vi "Sub_FFT.vi"(8 "Bound to 1st Frequency":bool=TRUE, 9 "Frequency Method":T2(ring), 10 "Accelerometer sample":dbl[](array[numeric]), 11 "Experiment":T1) -> (0 "Low-Energy Warning":bool, 1 "Frequency measured":dbl, 2 "FFT":dbl[](array[numeric]), 3 "ACC Data":dbl[](array[numeric]))   [LabVIEW 2021]
uses:
  <vilib>/Analysis/4window.llb/Hanning Window (DBL).vi
  <vilib>/Analysis/5stat.llb/RMS (DBL).vi
  <vilib>/Analysis/4window.llb/Hamming Window (DBL).vi
  <vilib>/Analysis/2dsp.llb/Real FFT.vi
  <vilib>/Analysis/4window.llb/AllCosWindow (DBL).vi
  <vilib>/addons/Time Series Analysis/Series Preprocess.llb/TSA Moving Average (Array).vi
  <vilib>/measure/maresamp.llb/Resample Waveform (continuous).vi
  <vilib>/Analysis/NI_AALPro.lvlib
  <vilib>/addons/_Advanced Signal Processing/NI_AdvSigProcTSA.lvlib
  <vilib>/measure/NI_MAPro.lvlib
panel:
  in  "Frequency selection method":T3(ring)
  in  "Use Top N freq components":i32=5 min=1 max=50 step=1
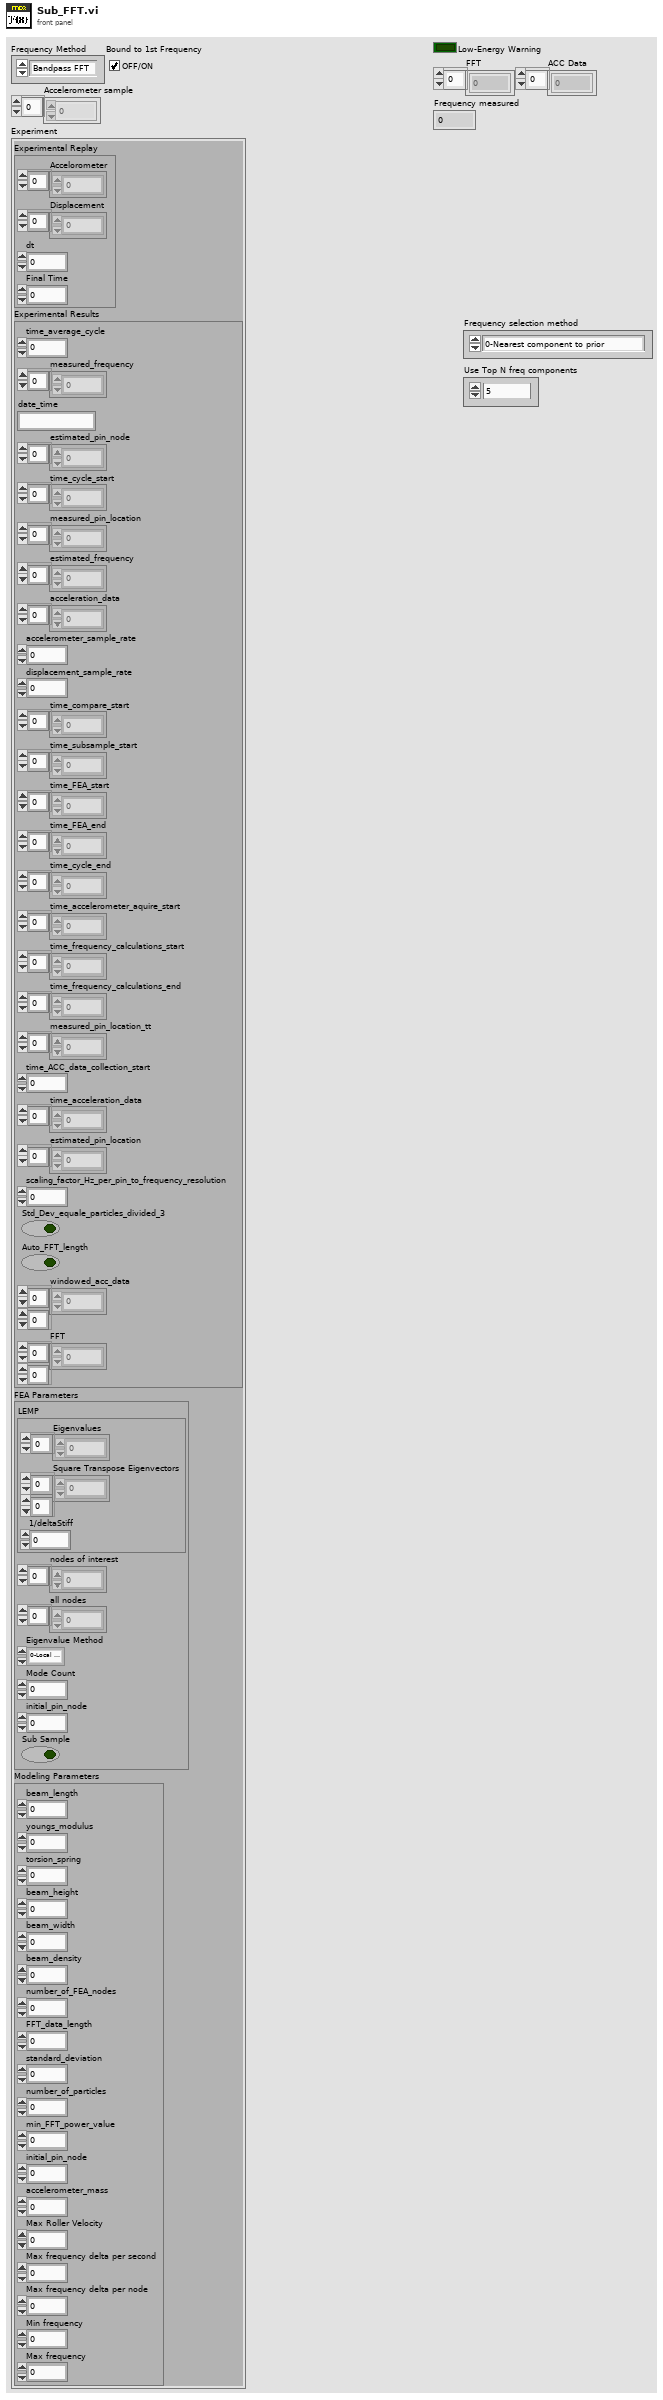
[diagram p1: front panel]
types:
  T1 = cluster{"Experimental Replay":cluster{"Accelorometer":dbl[], "Displacement":dbl[], "dt":dbl, "Final Time":dbl}, "Experimental Results":cluster{"time_average_cycle":dbl, "measured_frequency":dbl[], "date_time":string, "estimated_pin_node":i32[], "time_cycle_start":dbl[], "measured_pin_location":dbl[], "estimated_frequency":dbl[], "acceleration_data":dbl[], "accelerometer_sample_rate":dbl, "displacement_sample_rate":dbl, "time_compare_start":dbl[], "time_subsample_start":dbl[], "time_FEA_start":dbl[], "time_FEA_end":dbl[], "time_cycle_end":dbl[], "time_accelerometer_aquire_start":dbl[], "time_frequency_calculations_start":dbl[], "time_frequency_calculations_end":dbl[], "measured_pin_location_tt":dbl[], "time_ACC_data_collection_start":dbl, "time_acceleration_data":dbl[], "estimated_pin_location":dbl[], "scaling_factor_Hz_per_pin_to_frequency_resolution":dbl, "Std_Dev_equale_particles_divided_3":bool, "Auto_FFT_length":bool, "windowed_acc_data":dbl[][], "FFT":dbl[][]}, "FEA Parameters":cluster{"LEMP":cluster{"Eigenvalues":dbl[], "Square Transpose Eigenvectors":dbl[][], "1/deltaStiff":dbl}, "nodes of interest":i32[], "all nodes":i32[], "Eigenvalue Method":enum16{"0-Local Eigen Modification Procedure", "1-LabVIEW generalized eigenvalues", "2-LabVIEW M^-1K eigenvalues", "3-LabVIEW Cholesky Factorization", "4-Cholesky Factorization CPU SGL", "5-Cholesky Factorization CPU FXP", "6-Cholesky Factorization FPGA SGL", "7-Cholesky Factorization FPGA SGL SCL"}, "Mode Count":i32, "initial_pin_node":i32, "Sub Sample":bool}, "Modeling Parameters":cluster{"beam_length":dbl, "youngs_modulus":dbl, "torsion_spring":dbl, "beam_height":dbl, "beam_width":dbl, "beam_density":dbl, "number_of_FEA_nodes":i32, "FFT_data_length":i32, "standard_deviation":dbl, "number_of_particles":i32, "min_FFT_power_value":dbl, "initial_pin_node":i32, "accelerometer_mass":dbl, "Max Roller Velocity":dbl, "Max frequency delta per second":dbl, "Max frequency delta per node":dbl, "Min frequency":dbl, "Max frequency":dbl}}
  T2 = enum16{"Bandpass FFT", "Tone", "FFT", "Custom Filter"}
  T3 = enum16{"0-Nearest component to prior ", "1-Coerce maximum differential", "2-Average with nearest component", "3-Top by power", "4-Lowest major component", "5-Average with lowest component"}
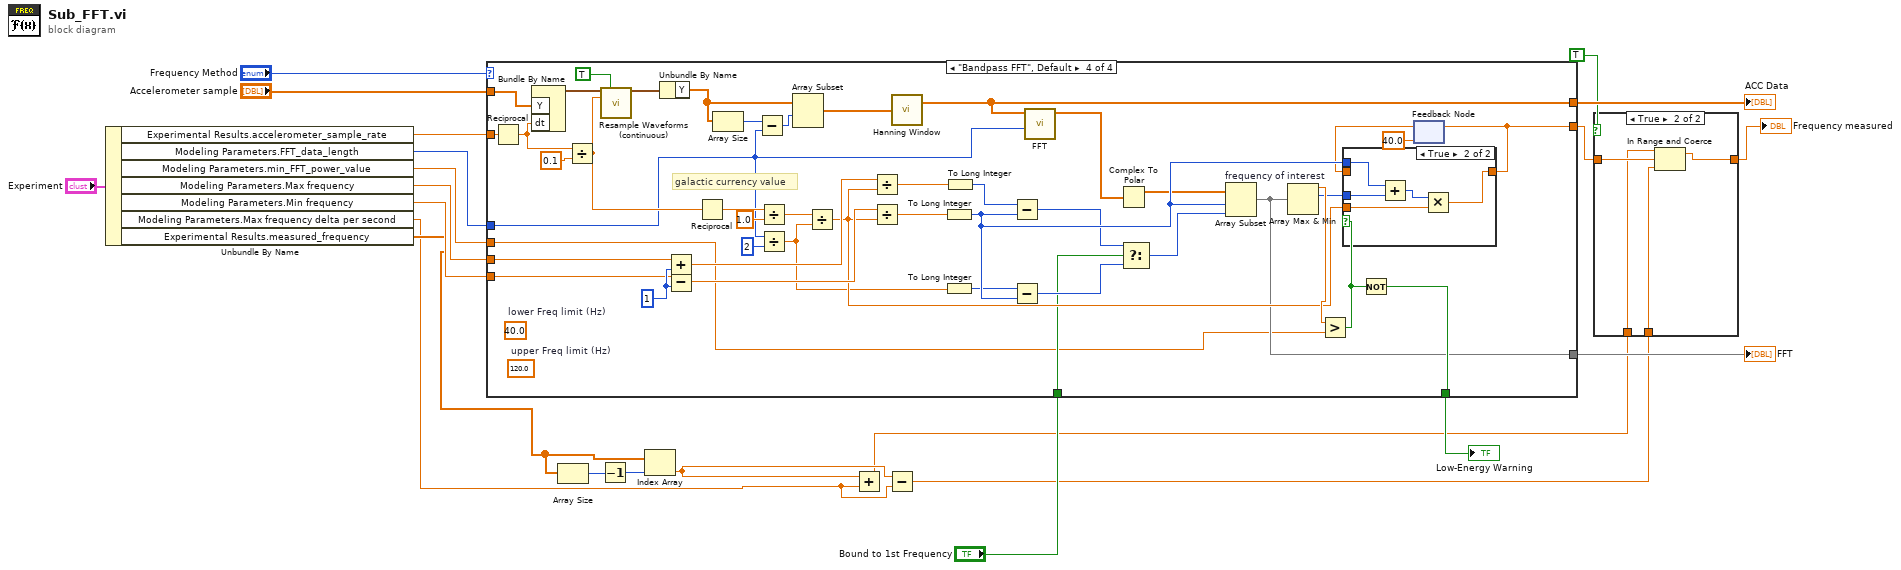
[diagram p0: block diagram]
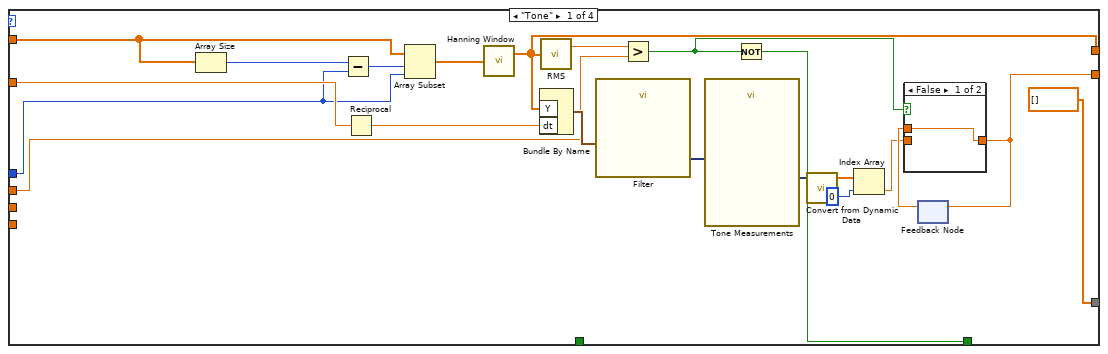
[diagram p3: hidden frame]
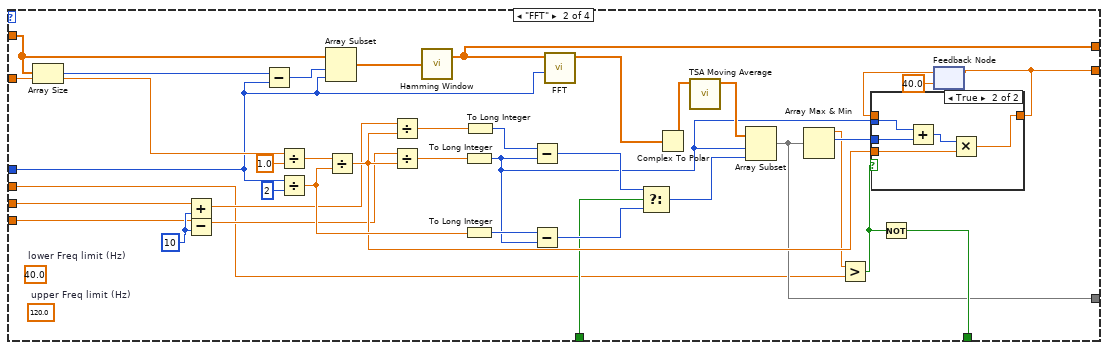
[diagram p5: hidden frame]
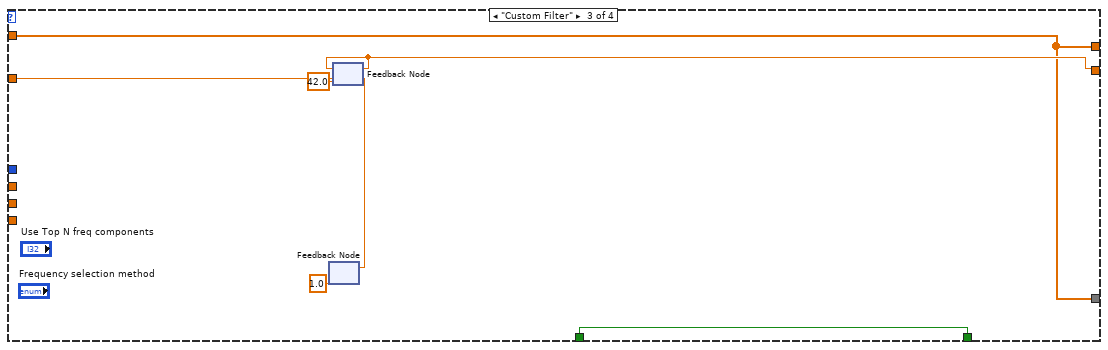
[diagram p7: hidden frame]
diagram:
  n1 = Unbundle By Name("Experiment") -> ("Experimental Results.accelerometer_sample_rate"=w19:dbl, "Modeling Parameters.FFT_data_length"=w15:i32, "Modeling Parameters.min_FFT_power_value"=w16:dbl, "Modeling Parameters.Max frequency"=w18:dbl, "Modeling Parameters.Min frequency"=w17:dbl, "Modeling Parameters.Max frequency delta per second"=w4:dbl, "Experimental Results.measured_frequency"=w8:dbl[])
  n2 = case shown="\"Bandpass FFT\", Default" "Frequency Method" {
    tunnel: [w31 w61 w95 w117] -> w10
    tunnel: [w33 w64 w90 w113] -> w11
    tunnel: "Accelerometer sample" -> [w35 w66 w90 w105]
    tunnel: [w28 w63 w94 w119] -> w13
    tunnel: "Bound to 1st Frequency" -> [_ w65 w94 w118]
    tunnel: [dbl[] [] ("Real freq comp (out)") w56 w90 w114] -> w12
    tunnel: w19 -> [w25 w50 w91 w110]
    tunnel: w18 -> [_ w47 _ w99]
    tunnel: w17 -> [_ w46 _ w98]
    tunnel: w16 -> [w23 w48 _ w97]
    tunnel: w15 -> [w24 w49 _ w96]
    frame "Tone" {
      n3 = Array Size(array=w35) -> (size(s)=w43:i32)
      n4 = Subtract(x=w43, y=w24) -> (x-y=w42:i32)
      n5 = Reciprocal(x=w25) -> (1/x=w27:dbl)
      n6 = Array Subset(array=w35, index=w42, length=w24) -> (w36:dbl[])
      n7 = call-poly <vilib>:"Hanning Window.vi"("X"=w36) -> ("Windowed X"=w33:dbl[])  [unwired: 1 out]
      n8 = Bundle By Name("Y"=w33, "dt"=w27) -> (w37:waveform(dbl))  [unwired: 1 in]
      n9 = call-poly <vilib>:"RMS.vi"("X"=w33) -> ("rms value"=w29:dbl)  [unwired: 1 out]
      n10 = call "Filter"("Signal"=w37) -> ("Filtered Signal"=w38:dynamicdata)  [unwired: 9 in, 1 out]
      n11 = Greater?(x=w29, y=w23) -> (0:w30:bool)
      n12 = call "Tone Measurements"("Signals"=w38) -> ("Frequency"=w39:dynamicdata)  [unwired: 9 in, 1 out]
      n13 = Not(x=w30) -> (.not. x?=w28:bool)
      n14 = call "Convert from Dynamic Data"("Dynamic Data Type"=w39) -> ("Array"=w40:dbl[])  [unwired: 3 in]
      n15 = Index Array(array=w40, index=0) -> (element=w32:dbl)
      n16 = feedback #1() -> (w34:dbl)  [unwired: 1 in]
      n17 = case shown="False" w30 {
        tunnel: [w44 w45] -> w31
        tunnel: w34 -> [w44 _]
        tunnel: w32 -> [_ w45]
        frame False {
        }
        frame True {
        }
      }
      n18 = feedback-in #1(w31) -> ()
    }
    frame "FFT" {
      w52 = 10
      (unwired) 120.0  # upper Freq limit (Hz)
      (unwired) 40.0  # lower Freq limit (Hz)
      n19 = Array Size(array=w66) -> (size(s)=w76:i32)
      n20 = Add(x=w47, y=w52) -> (x+y=w53:dbl)
      n21 = Subtract(x=w46, y=w52) -> (x-y=w54:dbl)
      n22 = Subtract(x=w76, y=w49) -> (x-y=w75:i32)
      n23 = Divide(x=w50, y=1.0) -> (x/y=w78:dbl)
      n24 = Divide(x=w49, y=2) -> (x/y=w77:dbl)
      n25 = Array Subset(array=w66, index=w75, length=w49) -> (w74:dbl[])
      n26 = Divide(x=w78, y=w77) -> (x/y=w72:dbl)
      n27 = Divide(x=w53, y=w72) -> (x/y=w71:dbl)
      n28 = Divide(x=w54, y=w72) -> (x/y=w82:dbl)
      n29 = call-poly <vilib>:"Hamming Window.vi"("X"=w74) -> ("Windowed X"=w64:dbl[])  [unwired: 1 out]
      n30 = To Long Integer(number=w82) -> (32bit integer=w55:i32)
      n31 = To Long Integer(number=w77) -> (32bit integer=w80:i32)
      n32 = To Long Integer(number=w71) -> (32bit integer=w70:i32)
      n33 = Subtract(x=w70, y=w55) -> (x-y=w68:i32)
      n34 = Subtract(x=w80, y=w55) -> (x-y=w67:i32)
      n35 = call-poly <vilib>:"FFT.vi"("FFT size"=w49, "X"=w64) -> ("FFT {X}"=w62:cdb[])  [unwired: 8 in, 1 out]
      n36 = Select(t=w68, s=w65, f=w67) -> (s? t:f=w69:i32)
      n37 = Complex To Polar(r * e^(i*theta)=w62) -> (r=w58:dbl[])  [unwired: 1 out]
      n38 = call-poly <vilib>:"TSA Moving Average.vi"("Xt"=w58) -> ("Xt out"=w57:dbl[])  [unwired: 9 in, 1 out]
      n39 = Array Subset(array=w57, index=w55, length=w69) -> (w56:dbl[])
      n40 = Array Max & Min(array=w56) -> (max value=w51:dbl, max index (indices)=w81:i32)  [unwired: 2 out]
      n41 = Greater?(x=w51, y=w48) -> (0:w73:bool)
      n42 = Not(x=w73) -> (.not. x?=w63:bool)
      n43 = feedback #2(40.0) -> (w60:dbl)
      n44 = case shown="True" w73 {
        tunnel: w81 -> [_ w85]
        tunnel: w55 -> [_ w86]
        tunnel: w72 -> [_ w87]
        tunnel: [w84 w88] -> w61
        tunnel: w60 -> [w84 _]
        frame False {
        }
        frame True {
          n45 = Add(x=w86, y=w85) -> (x+y=w89:i32)
          n46 = Multiply(x=w89, y=w87) -> (x*y=w88:dbl)
        }
      }
      n47 = feedback-in #2(w61) -> ()
    }
    frame "Custom Filter" {
      n48 = feedback #3(1.0 ("Slop factor (Feed back)")) -> ()  [unwired: 1 in]
      n49 = feedback-in #3(w91) -> ()
      n50 = feedback #4(42.0) -> (w95:dbl)
      n51 = feedback-in #4(w95) -> ()
    }
    frame "Bandpass FFT", Default {
      w120 = 1
      (unwired) 120.0  # upper Freq limit (Hz)
      (unwired) 40.0  # lower Freq limit (Hz)
      # "galactic currency value"
      n52 = Reciprocal(x=w110) -> (1/x=w109:dbl)
      n53 = Bundle By Name("Y"=w105, "dt"=w109) -> (w111:waveform(dbl))  [unwired: 1 in]
      n54 = Divide(x=w109, y=0.1) -> (x/y=w107:dbl)
      n55 = call-poly <vilib>:"Resample Waveforms (continuous).vi"("waveform in"=w111, "reset"=TRUE, "dt"=w107) -> ("resampled waveform out"=w112:waveform(dbl))  [unwired: 8 in, 4 out]
      n56 = Unbundle By Name(w112) -> ("Y"=w102:dbl[])
      n57 = Add(x=w99, y=w120) -> (x+y=w139:dbl)
      n58 = Subtract(x=w98, y=w120) -> (x-y=w138:dbl)
      n59 = Reciprocal(x=w107) -> (1/x=w106:dbl)
      n60 = Array Size(array=w102) -> (size(s)=w103:i32)
      n61 = Subtract(x=w103, y=w96) -> (x-y=w104:i32)
      n62 = Divide(x=w106, y=1.0) -> (x/y=w127:dbl)
      n63 = Divide(x=w96, y=2) -> (x/y=w128:dbl)
      n64 = Array Subset(array=w102, index=w104) -> (w101:dbl[])  [unwired: 1 in]
      n65 = Divide(x=w127, y=w128) -> (x/y=w130:dbl)
      n66 = Divide(x=w139, y=w130) -> (x/y=w131:dbl)
      n67 = Divide(x=w138, y=w130) -> (x/y=w124:dbl)
      n68 = call-poly <vilib>:"Hanning Window.vi"("X"=w101) -> ("Windowed X"=w113:dbl[])  [unwired: 1 out]
      n69 = To Long Integer(number=w124) -> (32bit integer=w137:i32)
      n70 = To Long Integer(number=w128) -> (32bit integer=w126:i32)
      n71 = To Long Integer(number=w131) -> (32bit integer=w132:i32)
      n72 = Subtract(x=w132, y=w137) -> (x-y=w134:i32)
      n73 = Subtract(x=w126, y=w137) -> (x-y=w135:i32)
      n74 = call-poly <vilib>:"FFT.vi"("FFT size"=w96, "X"=w113) -> ("FFT {X}"=w116:cdb[])  [unwired: 8 in, 1 out]
      n75 = Complex To Polar(r * e^(i*theta)=w116) -> (r=w115:dbl[])  [unwired: 1 out]
      n76 = Select(t=w134, s=w118, f=w135) -> (s? t:f=w133:i32)
      n77 = Array Subset "frequency of interest"(array=w115, index=w137, length=w133) -> (w114:dbl[])
      n78 = Array Max & Min(array=w114) -> (max value=w140:dbl, max index (indices)=w125:i32)  [unwired: 2 out]
      n79 = Greater?(x=w140, y=w97) -> (0:w129:bool)
      n80 = Not(x=w129) -> (.not. x?=w119:bool)
      n81 = feedback #5(40.0) -> (w136:dbl)
      n82 = case shown="True" w129 {
        tunnel: w125 -> [_ w142]
        tunnel: w137 -> [_ w143]
        tunnel: w130 -> [_ w144]
        tunnel: [w141 w145] -> w117
        tunnel: w136 -> [w141 _]
        frame False {
        }
        frame True {
          n83 = Add(x=w143, y=w142) -> (x+y=w146:i32)
          n84 = Multiply(x=w146, y=w144) -> (x*y=w145:dbl)
        }
      }
      n85 = feedback-in #5(w117) -> ()
    }
  }
  "Low-Energy Warning" <- w13
  "FFT" <- w12
  "ACC Data" <- w11
  n86 = Array Size(array=w8) -> (size(s)=w7:i32)
  n87 = Decrement(x=w7) -> (x-1=w6:i32)
  n88 = Index Array(array=w8, index=w6) -> (element=w5:dbl)
  n89 = Add(x=w5, y=w4) -> (x+y=w3:dbl)
  n90 = Subtract(x=w5, y=w4) -> (x-y=w2:dbl)
  n91 = case shown="True" TRUE {
    tunnel: w10 -> [w147 w151]
    tunnel: [w147 w150] -> w9
    tunnel: w3 -> [_ w149]
    tunnel: w2 -> [_ w148]
    frame False {
    }
    frame True {
      n92 = In Range and Coerce(upper limit=w149, x=w151, lower limit=w148) -> (coerced(x)=w150:dbl)  [unwired: 1 out]
    }
  }
  "Frequency measured" <- w9
